vi "Read Type (Pub, Sub).vi"(8 "error in (no error)":errorcluster, 11 "ZMQ in":refnum<class "ZMQ.lvclass">) -> (0 "error out":errorcluster, 2 "Type (Pub, Sub)":T1, 3 "ZMQ out":refnum<class "ZMQ.lvclass">)   [LabVIEW 2016]
uses:
  ZMQ.lvclass
  C:/Program Files (x86)/National Instruments/LabVIEW 2016/vi.lib/JKI/JKI SMO/SMO/SMO.lvclass
  Typedefs/ZMQ Type -- Typedef.ctl
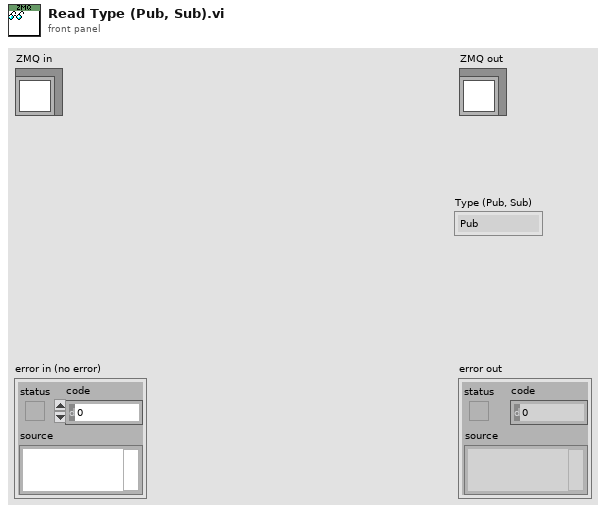
[diagram p1: front panel]
types:
  T1 = typedef "ZMQ.lvclass/ZMQ Type -- Typedef.ctl" = enum16{"Pub", "Sub", "Rep"}
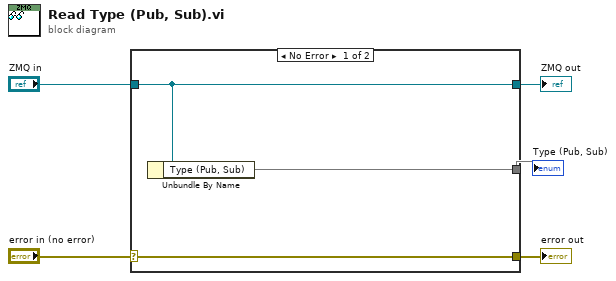
[diagram p0: block diagram]
diagram:
  n1 = case shown="No Error" "error in (no error)" {
    selector: "error in (no error)" -> [w8 w9]
    tunnel: [w8 w9] -> w4
    tunnel: [w7 w10] -> w2
    tunnel: "ZMQ in" -> [w7 w10]
    tunnel: [w6 _] -> w1
    frame No Error {
      n2 = Unbundle By Name(w7) -> ("Type (Pub, Sub)"=w6)
    }
    frame Error {
    }
  }
  "error out" <- w4
  "ZMQ out" <- w2
  "Type (Pub, Sub)" <- w1
